vi "Msg To.vi"() -> (3 "Pop Up Msg Strategy out":refnum<class "Pop Up Msg Strategy.lvclass">)   [LabVIEW 2021, in "Pop Up.lvlib" / "Pop Up Msg Strategy.lvclass"]
uses:
  Pop Up Msg Strategy.lvclass
  Pop Up Msg Strategy.lvclass/Pop Up Msg Strategy.ctl
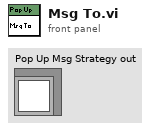
[diagram p1: front panel]
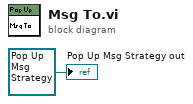
[diagram p0: block diagram]
diagram:
  "Pop Up Msg Strategy out" <- refnum<class "Pop Up Msg Strategy.lvclass"> refnum ("Pop Up Msg Strategy out")
